vi "USBInit.vi"(4 "error in (no error)":errorcluster, 6 "Product ID":string, 7 "logging":bool) -> (0 "error out":errorcluster, 2 "Pass-Fail Status":bool, 3 "USBLib Out":refnum<k24>)   [LabVIEW 2009]
uses:
  C:/Samples/LabVIEW/UseDeviceKey/LabVIEW 2009/UseDeviceKey (with Device VIs)/UsbDllWrap.dll
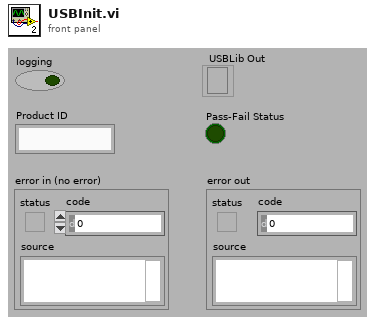
[diagram p1: front panel]
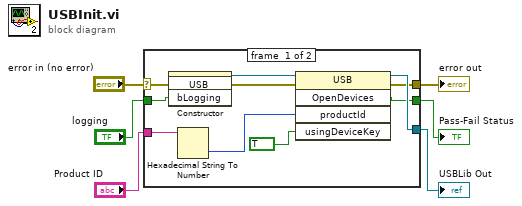
[diagram p0: block diagram]
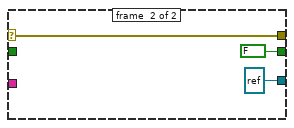
[diagram p2: hidden frame]
diagram:
  n1 = case shown="No Error" "error in (no error)" {
    selector: "error in (no error)" -> [w7 w17]
    tunnel: "logging" -> [w16 _]
    tunnel: [w13 refnum<k24> refnum ("new reference")] -> w5
    tunnel: [w12 FALSE ("OpenDevices")] -> w4
    tunnel: "Product ID" -> [w9 _]
    tunnel: [w8 w17] -> w1
    frame #0 {
      n2 = constructor class="USB"(error in=w7, "bLogging"=w16) -> (reference out=w15:refnum<k24>, error out=w14:errorcluster)  [unwired: 2 in, 2 out]
      n3 = Hexadecimal String To Number(string=w9) -> (number=w11:u32)  [unwired: 2 in, 1 out]
      n4 = invoke class="USB" method="OpenDevices"(reference=w15, error in=w14, "productId"=w11, "usingDeviceKey"=TRUE) -> (reference out=w13:refnum<k24>, error out=w8:errorcluster, "OpenDevices"=w12:bool)  [unwired: 1 in, 2 out]
    }
    frame #1 {
    }
  }
  "error out" <- w1
  "USBLib Out" <- w5
  "Pass-Fail Status" <- w4
